vi "Data_Save_good.vi"(9 "Data":T1) -> (2 "good":string[](array[string]))   [LabVIEW 2017]
uses:
  Ctrls/Data.ctl
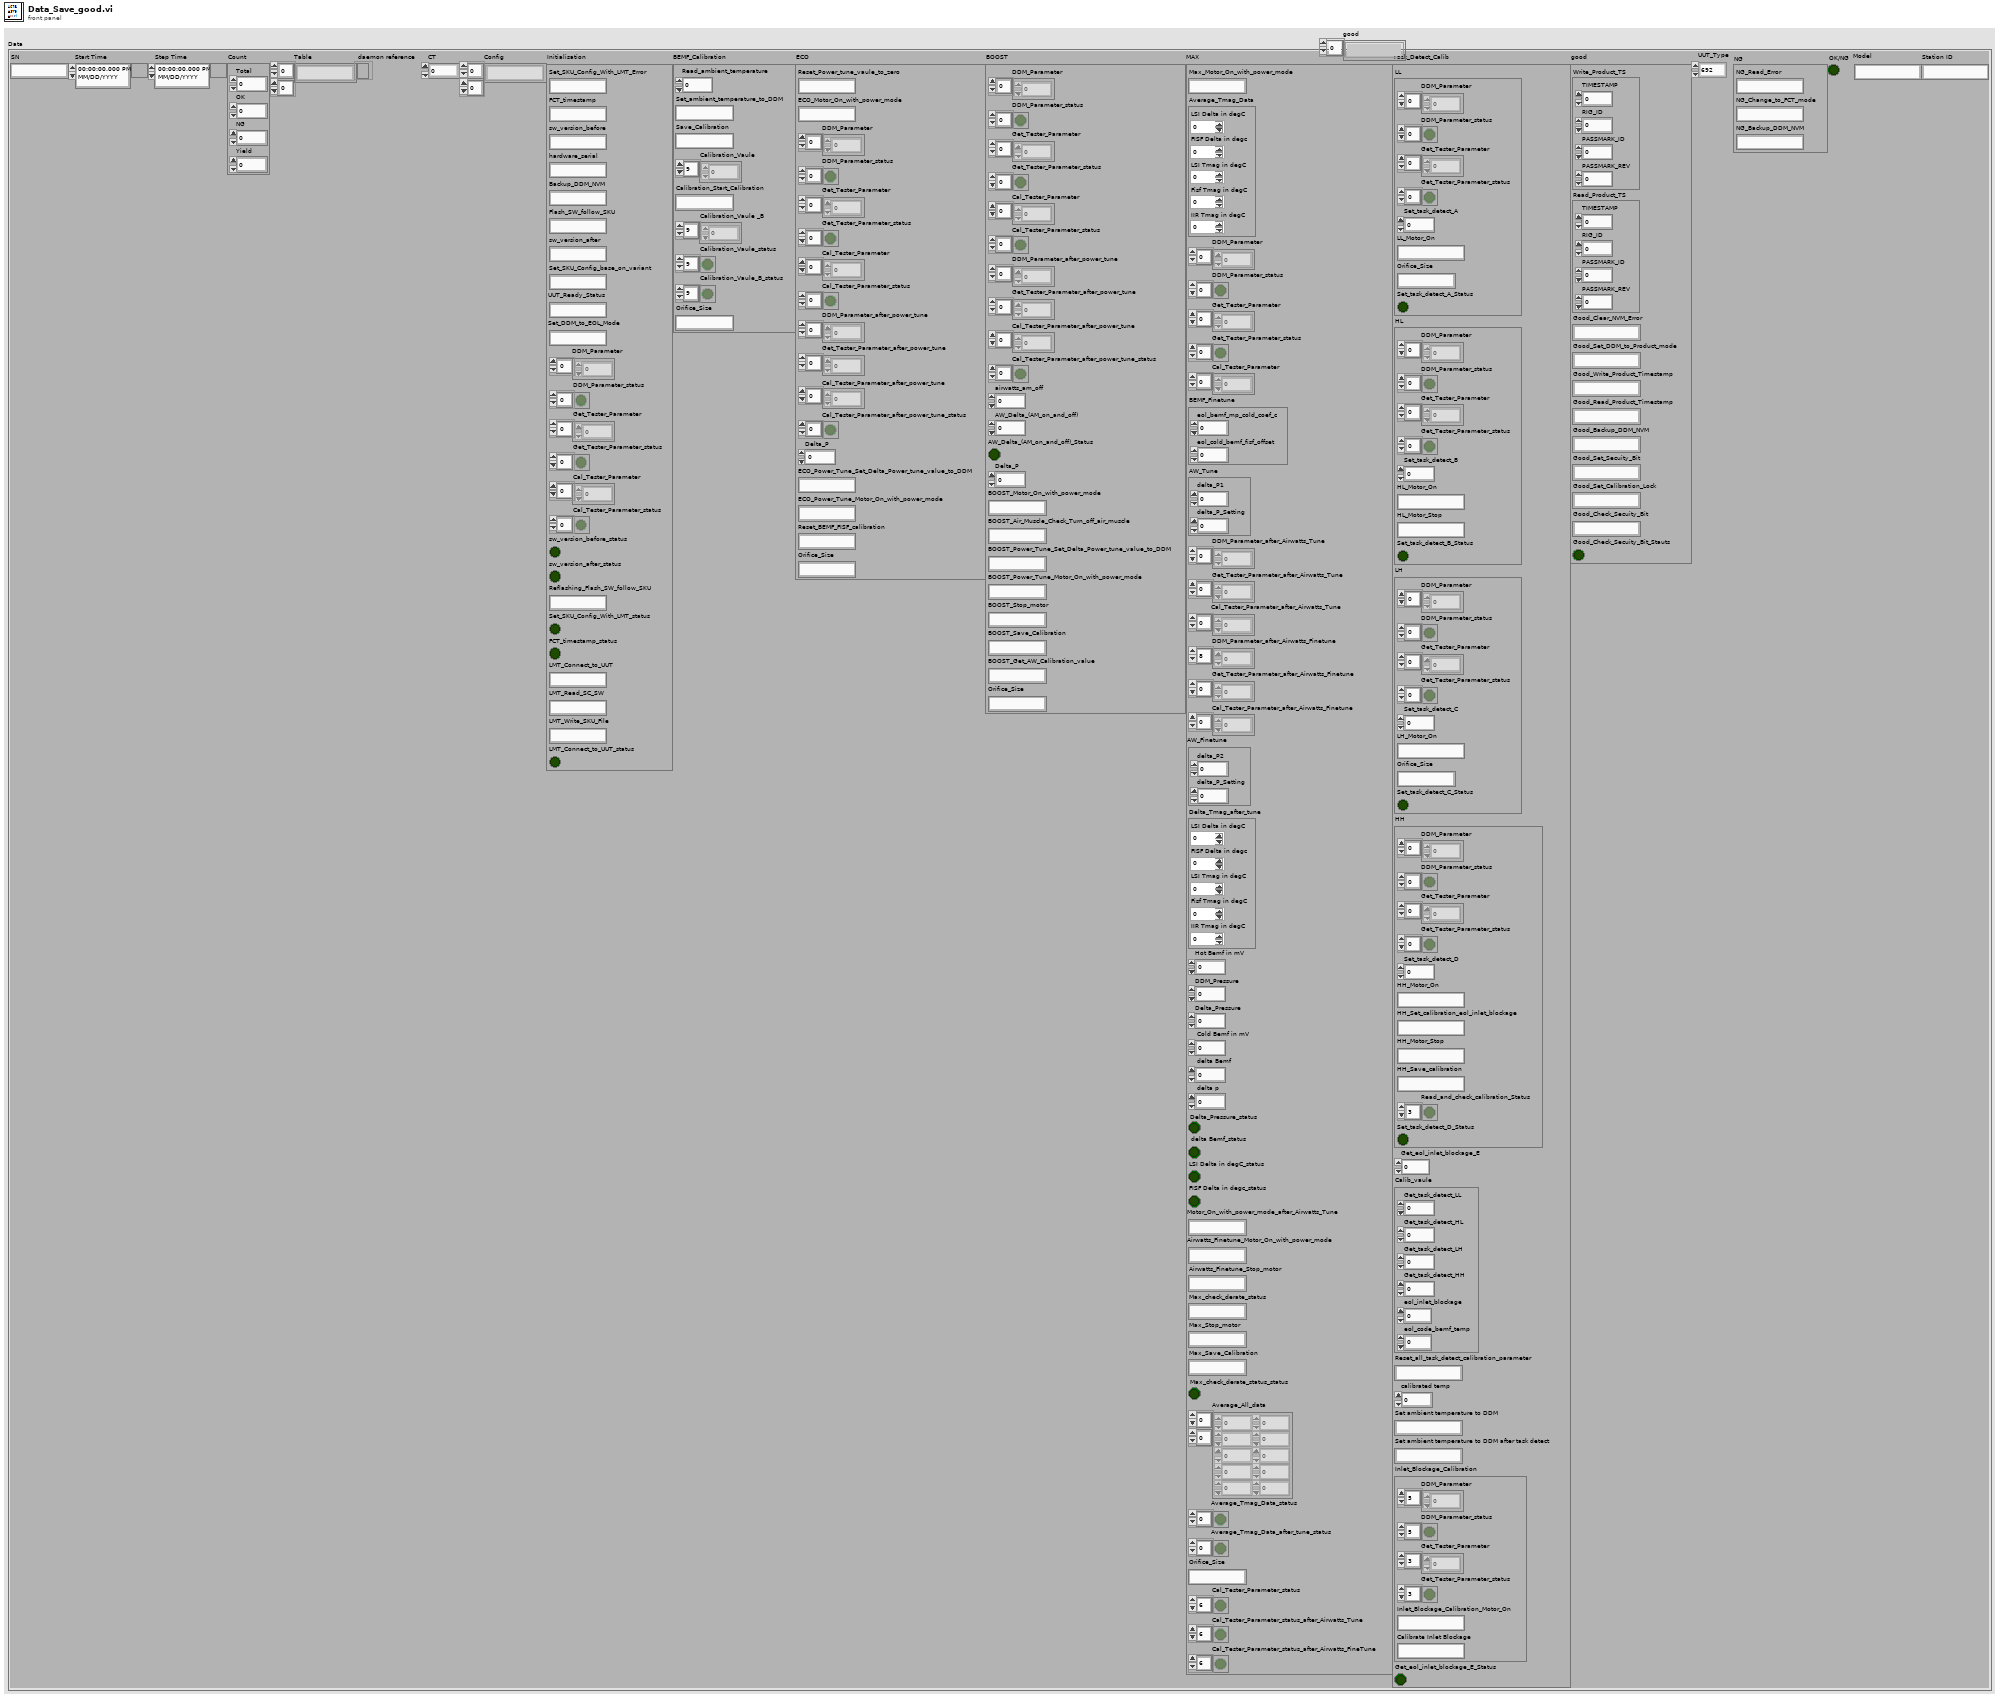
[diagram p1: front panel]
types:
  T1 = typedef "Data.ctl" = cluster{"SN":string, "Start Time":timestamp, "Step Time":timestamp, "Count":cluster{"Total":i32, "OK":i32, "NG":i32, "Yield":dbl}, "Table":string[][], "daemon reference":refnum<k5>, "CT":dbl, "Config":string[][], "Initialisation":cluster{"Set_SKU_Config_With_LMT_Error":string, "FCT_timestamp":string, "sw_version_before":string, "hardware_serial":string, "Backup_DDM_NVM":string, "Flash_SW_follow_SKU":string, "sw_version_after":string, "Set_SKU_Config_base_on_variant":string, "UUT_Ready_Status":string, "Set_DDM_to_EOL_Mode":string, "DDM_Parameter":dbl[], "DDM_Parameter_status":bool[], "Get_Tester_Parameter":dbl[], "Get_Tester_Parameter_status":bool[], "Cal_Tester_Parameter":dbl[], "Cal_Tester_Parameter_status":bool[], "sw_version_before_status":bool, "sw_version_after_status":bool, "Reflashing_Flash_SW_follow_SKU":string, "Set_SKU_Config_With_LMT_status":bool, "FCT_timestamp_status":bool, "LMT_Connect_to_UUT":string, "LMT_Read_SC_SW":string, "LMT_Write_SKU_File":string, "LMT_Connect_to_UUT_status":bool}, "BEMF_Calibration":cluster{"Read_ambient_temperature":dbl, "Set_ambient_temperature_to_DDM":string, "Save_Calibration":string, "Calibration_Vaule":dbl[], "Calibration_Start_Calibration":string, "Calibration_Vaule _B":dbl[], "Calibration_Vaule_status":bool[], "Calibration_Vaule_B_status":bool[], "Orifice_Size":string}, "ECO":cluster{"Reset_Power_tune_vaule_to_zero":string, "ECO_Motor_On_with_power_mode":string, "DDM_Parameter":dbl[], "DDM_Parameter_status":bool[], "Get_Tester_Parameter":dbl[], "Get_Tester_Parameter_status":bool[], "Cal_Tester_Parameter":dbl[], "Cal_Tester_Parameter_status":bool[], "DDM_Parameter_after_power_tune":dbl[], "Get_Tester_Parameter_after_power_tune":dbl[], "Cal_Tester_Parameter_after_power_tune":dbl[], "Cal_Tester_Parameter_after_power_tune_status":bool[], "Delta_P":dbl, "ECO_Power_Tune_Set_Delta_Power_tune_value_to_DDM":string, "ECO_Power_Tune_Motor_On_with_power_mode":string, "Reset_BEMF_FISF_calibration":string, "Orifice_Size":string}, "BOOST":cluster{"DDM_Parameter":dbl[], "DDM_Parameter_status":bool[], "Get_Tester_Parameter":dbl[], "Get_Tester_Parameter_status":bool[], "Cal_Tester_Parameter":dbl[], "Cal_Tester_Parameter_status":bool[], "DDM_Parameter_after_power_tune":dbl[], "Get_Tester_Parameter_after_power_tune":dbl[], "Cal_Tester_Parameter_after_power_tune":dbl[], "Cal_Tester_Parameter_after_power_tune_status":bool[], "airwatts_am_off":dbl, "AW_Delta_(AM_on_and_off)":dbl, "AW_Delta_(AM_on_and_off)_Status":bool, "Delta_P":dbl, "BOOST_Motor_On_with_power_mode":string, "BOOST_Air_Muscle_Check_Turn_off_air_muscle":string, "BOOST_Power_Tune_Set_Delta_Power_tune_value_to_DDM":string, "BOOST_Power_Tune_Motor_On_with_power_mode":string, "BOOST_Stop_motor":string, "BOOST_Save_Calibration":string, "BOOST_Get_AW_Calibration_value":string, "Orifice_Size":string}, "MAX":cluster{"Max_Motor_On_with_power_mode":string, "Average_Tmag_Data":cluster{"LSI Delta in degC":dbl, "FISF Delta in degc":dbl, "LSI Tmag in degC":dbl, "Fisf Tmag in degC":dbl, "IIR Tmag in degC":dbl}, "DDM_Parameter":dbl[], "DDM_Parameter_status":bool[], "Get_Tester_Parameter":dbl[], "Get_Tester_Parameter_status":bool[], "Cal_Tester_Parameter":dbl[], "BEMF_Finetune":cluster{"eol_bemf_mp_cold_coef_c":dbl, "eol_cold_bemf_fisf_offset":dbl}, "AW_Tune":cluster{"delta_P1":dbl, "delta_P_Setting":dbl}, "DDM_Parameter_after_Airwatts_Tune":dbl[], "Get_Tester_Parameter_after_Airwatts_Tune":dbl[], "Cal_Tester_Parameter_after_Airwatts_Tune":dbl[], "DDM_Parameter_after_Airwatts_Finetune":dbl[], "Get_Tester_Parameter_after_Airwatts_Finetune":dbl[], "Cal_Tester_Parameter_after_Airwatts_Finetune":dbl[], "AW_Finetune":cluster{"delta_P2":dbl, "delta_P_Setting":dbl}, "Delta_Tmag_after_tune":cluster{"LSI Delta in degC":dbl, "FISF Delta in degc":dbl, "LSI Tmag in degC":dbl, "Fisf Tmag in degC":dbl, "IIR Tmag in degC":dbl}, "Hot Bemf in mV":dbl, "DDM_Pressure":dbl, "Delta_Pressure":dbl, " Cold Bemf in mV":dbl, " delta Bemf":dbl, " delta p":dbl, "Delta_Pressure_status":bool, " delta Bemf_status":bool, "LSI Delta in degC_status":bool, "FISF Delta in degc_status":bool, "Motor_On_with_power_mode_after_Airwatts_Tune":string, "Airwatts_Finetune_Motor_On_with_power_mode":string, "Airwatts_Finetune_Stop_motor":string, "Max_check_derate_status":string, "Max_Stop_motor":string, "Max_Save_Calibration":string, "Max_check_derate_status_status":bool, "Average_All_data":dbl[][], "Average_Tmag_Data_status":bool[], "Average_Tmag_Data_after_tune_status":bool[], "Orifice_Size":string, "Cal_Tester_Parameter_status":bool[], "Cal_Tester_Parameter_status_after_Airwatts_Tune":bool[], "Cal_Tester_Parameter_status_after_Airwatts_FineTune":bool[]}, "Task_Detect_Calib":cluster{"LL":cluster{"DDM_Parameter":dbl[], "DDM_Parameter_status":bool[], "Get_Tester_Parameter":dbl[], "Get_Tester_Parameter_status":bool[], "Set_task_detect_A":dbl, "LL_Motor_On":string, "Orifice_Size":string, "Set_task_detect_A_Status":bool}, "HL":cluster{"DDM_Parameter":dbl[], "DDM_Parameter_status":bool[], "Get_Tester_Parameter":dbl[], "Get_Tester_Parameter_status":bool[], "Set_task_detect_B":dbl, "HL_Motor_On":string, "HL_Motor_Stop":string, "Set_task_detect_B_Status":bool}, "LH":cluster{"DDM_Parameter":dbl[], "DDM_Parameter_status":bool[], "Get_Tester_Parameter":dbl[], "Get_Tester_Parameter_status":bool[], "Set_task_detect_C":dbl, "LH_Motor_On":string, "Orifice_Size":string, "Set_task_detect_C_Status":bool}, "HH":cluster{"DDM_Parameter":dbl[], "DDM_Parameter_status":bool[], "Get_Tester_Parameter":dbl[], "Get_Tester_Parameter_status":bool[], "Set_task_detect_D":dbl, "HH_Motor_On":string, "HH_Set_calibration_eol_inlet_blockage":string, "HH_Motor_Stop":string, "HH_Save_calibration":string, "Read_and_check_calibration_Status":bool[], "Set_task_detect_D_Status":bool}, "Get_eol_inlet_blockage_E":dbl, "Calib_vaule":cluster{"Get_task_detect_LL":dbl, "Get_task_detect_HL":dbl, "Get_task_detect_LH":dbl, "Get_task_detect_HH":dbl, "eol_inlet_blockage":dbl, "eol_code_bemf_temp":dbl}, "Reset_all_task_detect_calibration_parameter":string, "calibrated temp":dbl, "Set ambient temperature to DDM":string, "Set ambient temperature to DDM after task detect":string, "Inlet_Blockage_Calibration":cluster{"DDM_Parameter":dbl[], "DDM_Parameter_status":bool[], "Get_Tester_Parameter":dbl[], "Get_Tester_Parameter_status":bool[], "Inlet_Blockage_Calibration_Motor_On":string, "Calibrate Inlet Blockage":string}, "Get_eol_inlet_blockage_E_Status":bool}, "good":cluster{"Write_Product_TS":cluster{"TIMESTAMP":i64, "RIG_ID":i64, "PASSMARK_ID":i64, "PASSMARK_REV":i64}, "Read_Product_TS":cluster{"TIMESTAMP":i64, "RIG_ID":i64, "PASSMARK_ID":i64, "PASSMARK_REV":i64}, "Good_Clear_NVM_Error":string, "Good_Set_DDM_to_Product_mode":string, "Good_Write_Product_Timestamp":string, "Good_Read_Product_Timestamp":string, "Good_Backup_DDM_NVM":string, "Good_Set_Secuity_Bit":string, "Good_Set_Calibration_Lock":string, "Good_Check_Secuity_Bit":string, "Good_Check_Secuity_Bit_Stauts":bool}, "UUT_Type":enum16{"692", "692B", "692D"}, "NG":cluster{"NG_Read_Error":string, "NG_Change_to_FCT_mode":string, "NG_Backup_DDM_NVM":string}, "OK/NG":bool, "Model":string, "Station ID":string}
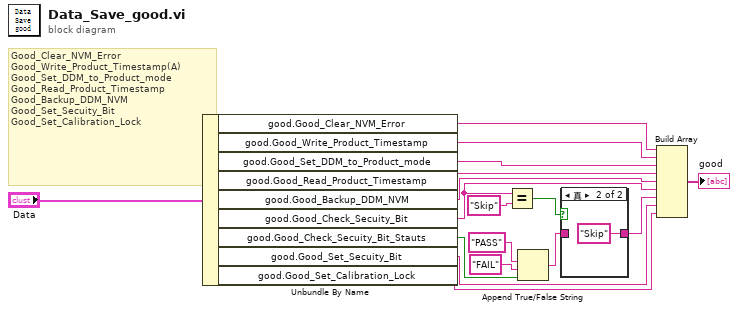
[diagram p0: block diagram]
diagram:
  # "Good_Clear_NVM_Error\nGood_Write_Product_Timestamp(A)\nGood_Set_DDM_to_Product_mode\nGood_Read_Product_Timestamp\nGood_Backup_DDM_NVM\nGood_Set_Secuity_Bit\nGood_Set_Calibration_Lock"
  n1 = Unbundle By Name("Data") -> ("good.Good_Clear_NVM_Error"=w1:string, "good.Good_Write_Product_Timestamp"=w15:string, "good.Good_Set_DDM_to_Product_mode"=w14:string, "good.Good_Read_Product_Timestamp"=w13:string, "good.Good_Backup_DDM_NVM"=w12:string, "good.Good_Check_Secuity_Bit"=w3:string, "good.Good_Check_Secuity_Bit_Stauts"=w4:bool, "good.Good_Set_Secuity_Bit"=w11:string, "good.Good_Set_Calibration_Lock"=w10:string)
  n2 = Equal?(x=w3, y="Skip" ("x")) -> (x = y?=w6:bool)
  n3 = Append True/False String(1:w4, 2:"FAIL" ("字符串(\"\")"), 3:"PASS" ("真字符串")) -> (0:w5:string)  [unwired: 1 in]
  n4 = case shown="真" w6 {
    tunnel: [w18 "Skip" ("x")] -> w2
    tunnel: w5 -> [w18 _]
    frame False {
    }
    frame True {
    }
  }
  n5 = Build Array(w1, w15, w14, w13, w12, w3, w2, w11, w10) -> (→"good":string[])
